vi "CRYUnflatten Display.vi"(11 "Flatten Display":string) -> (0 "Error?":bool=TRUE, 2 "DataView GUI Info":T1, 3 "Header info":T2={"Data type"="Data            ", "Version"=1, "Dimensions"=0})   [LabVIEW 2013]
uses:
  CRYWindow/DataView/VIEW/Control/Graph Main Info Cluster.ctl
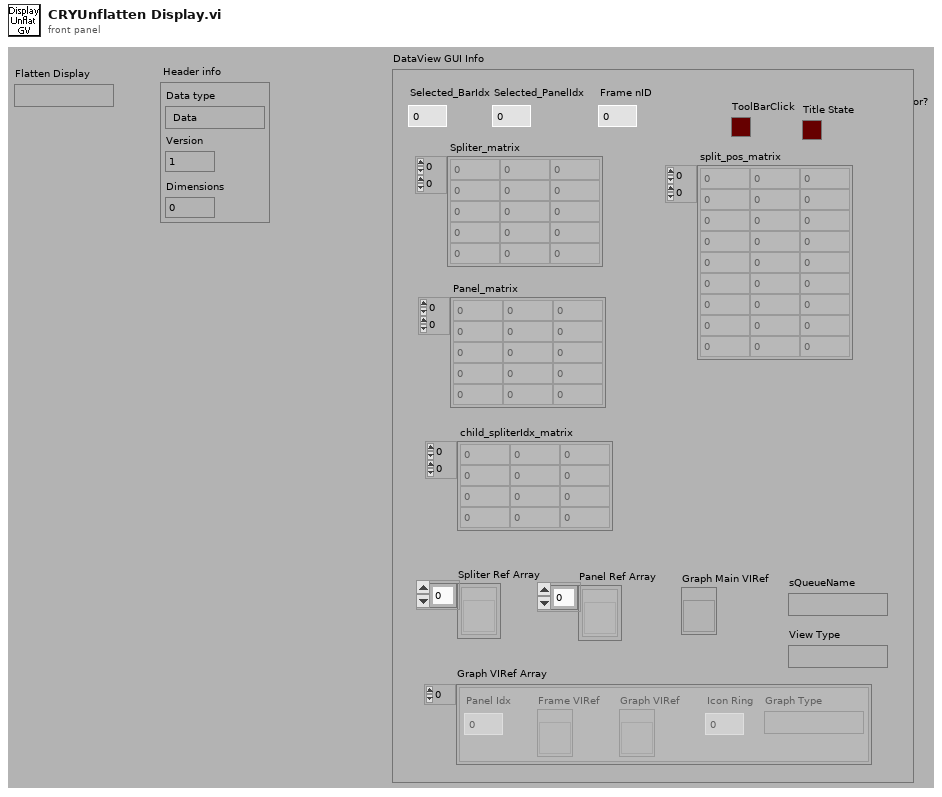
[diagram p1: front panel]
types:
  T1 = typedef "Graph Main Info Cluster.ctl" = cluster{"Selected_BarIdx":i32, "Selected_PanelIdx":i32, "Graph Main VIRef":refnum<vi>, "ToolBarClick":bool, "Spliter Ref Array":refnum<vi>[], "Panel Ref Array":refnum<vi>[], "Spliter_matrix":i32[][], "Panel_matrix":i32[][], "child_spliterIdx_matrix":i32[][], "split_pos_matrix":i32[][], "Title State":bool, "sQueueName":string, "Frame nID":i32, "Graph VIRef Array":cluster{"Graph VIRef":refnum<vi>, "Panel Idx":i32, "Frame VIRef":refnum<vi>, "Icon Ring":i32, "Graph Type":string}[], "View Type":string}
  T2 = cluster{"Data type":string, "Version":u16, "Dimensions":u8}
  T3 = cluster{"unsigned byte array[0]":u8, "unsigned byte array[1]":u8, "unsigned byte array[2]":u8}
  T4 = cluster{"substring":string, u16, "unsigned byte array[2]":u8}
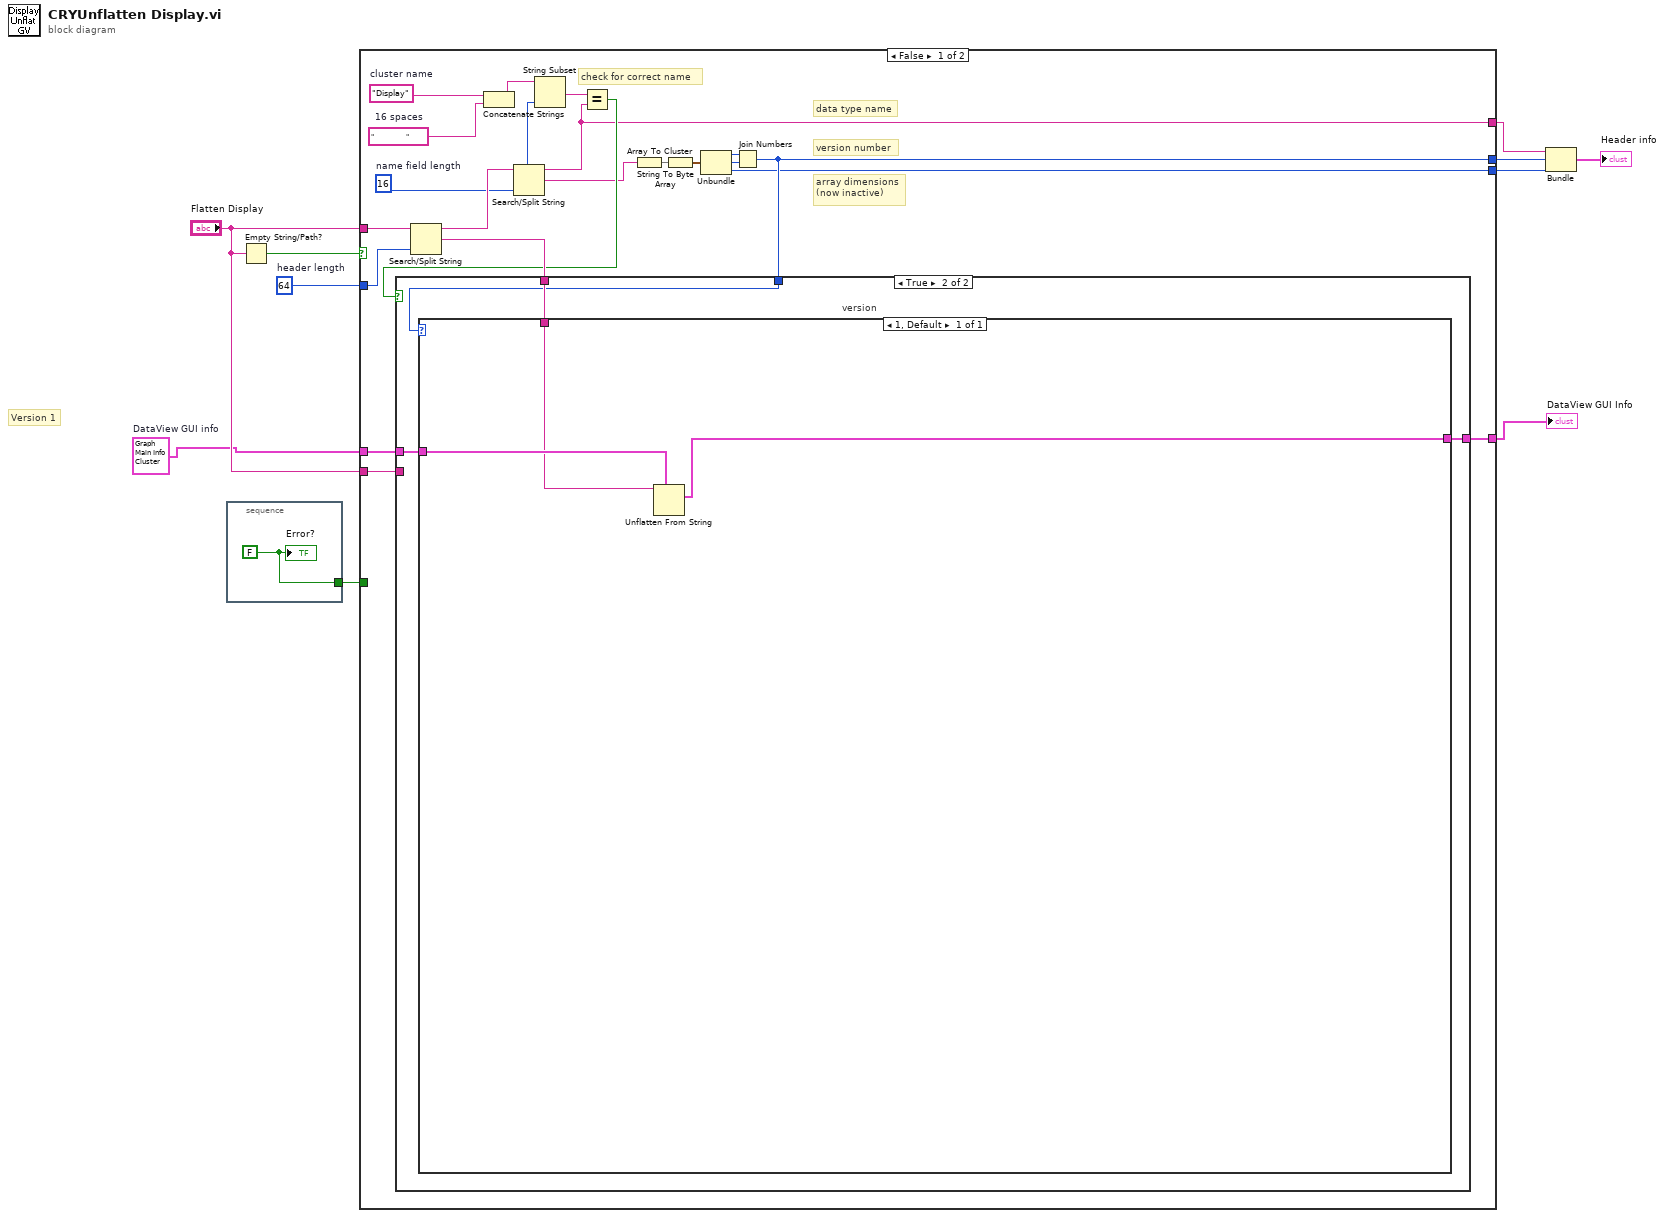
[diagram p0: block diagram]
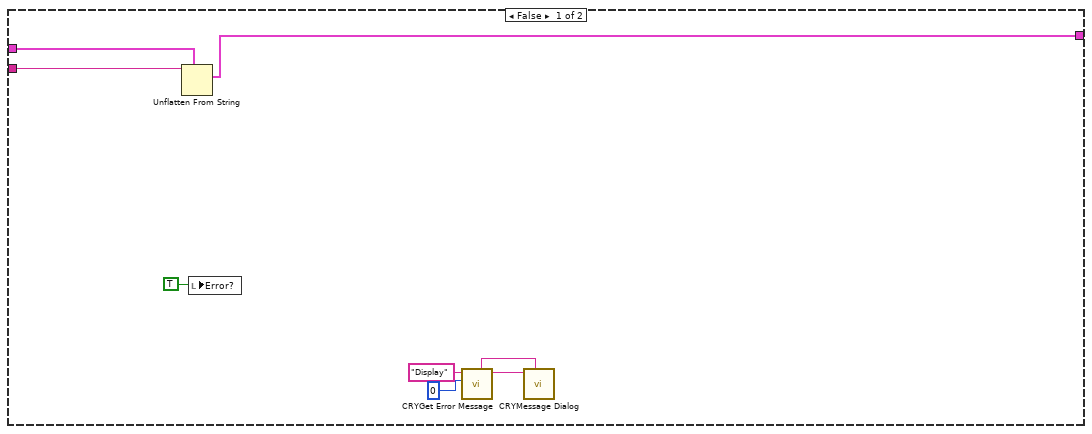
[diagram p2: hidden frame]
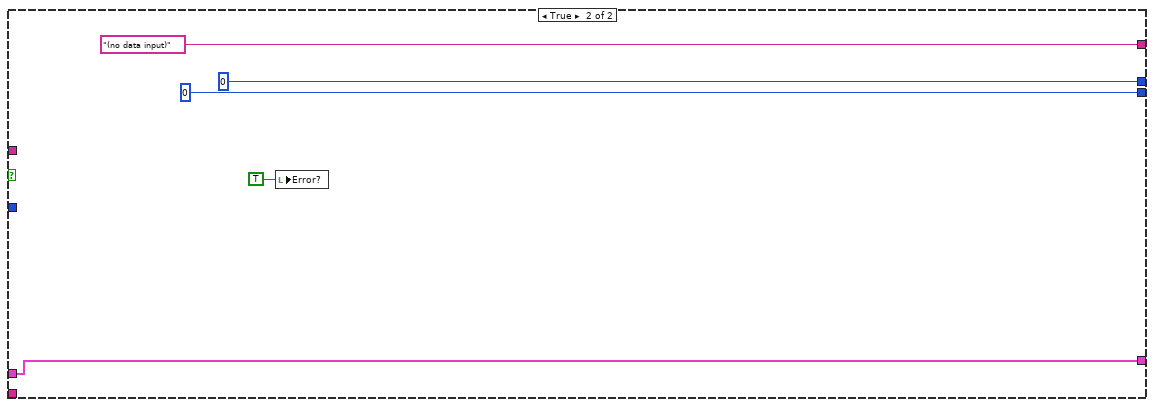
[diagram p3: hidden frame]
diagram:
  w2 = T1 {"Selected_BarIdx"=0, "Selected_PanelIdx"=0, "Graph Main VIRef"=refnum, "ToolBarClick"=FALSE, "Spliter Ref Array"=[], "Panel Ref Array"=[], "Spliter_matrix"=[], "Panel_matrix"=[], "child_spliterIdx_matrix"=[], "split_pos_matrix"=[], "Title State"=FALSE, "sQueueName"="", "Frame nID"=0, "Graph VIRef Array"=[], "View Type"=""}  # DataView GUI info
  w9 = 64  # header length
  # "Version 1"
  n1 = stacked-sequence {
    tunnel: [w11] -> w4
    frame #0 {
      w11 = FALSE
      "Error?" <- w11
    }
  }
  n2 = Empty String/Path?(string/path="Flatten Display") -> (empty?=w10:bool)
  n3 = case shown="False" w10 {
    tunnel: "Flatten Display" -> [w32 _]
    tunnel: w9 -> [w26 _]
    tunnel: [w23 u16 0] -> w7
    tunnel: [w15 u8 0] -> w8
    tunnel: [w16 "(no data input)" ("substring")] -> w6
    tunnel: w4 -> [_ _]
    tunnel: [w14 w48] -> w1
    tunnel: w2 -> [w13 w48]
    tunnel: "Flatten Display" -> [w12 _]
    frame False {
      w20 = "                "  # 16 spaces
      w21 = "Display"  # cluster name
      w18 = 16  # name field length
      # "check for correct name"
      # "array dimensions\n(now inactive)"
      # "version number"
      # "data type name"
      n4 = Search/Split String(string=w32, offset (0)=w26) -> (substring before match=w25:string, match + rest of string=w27:string)  [unwired: 2 out]
      n5 = Concatenate Strings(w21, w20) -> (w19:string)
      n6 = Search/Split String(string=w25, offset (0)=w18) -> (substring before match=w16:string, match + rest of string=w22:string)  [unwired: 2 out]
      n7 = String Subset(string=w19, length (rest)=w18) -> (substring=w17:string)  [unwired: 1 out]
      n8 = Equal?(x=w17, y=w16) -> (x = y?=w24:bool)
      n9 = String To Byte Array(string=w22) -> (unsigned byte array=w31:u8[])
      n10 = Array To Cluster(array=w31) -> (cluster=w30:T3)
      n11 = Unbundle(w30) -> ("unsigned byte array[0]"=w29:u8, "unsigned byte array[1]"=w28:u8, "unsigned byte array[2]"=w15:u8)
      n12 = Join Numbers(hi=w29, lo=w28) -> ((hi.lo)=w23:u16)
      n13 = case shown="True" w24 {
        tunnel: w27 -> [_ w44]
        tunnel: w23 -> [_ w43]
        tunnel: [w38 w41] -> w14
        tunnel: w13 -> [w39 w42]
        tunnel: w12 -> [w37 _]
        frame False {
          n14 = Unflatten From String(type=w39, binary string=w37) -> (value=w38:T1)  [unwired: 3 in, 2 out]
          n15 = local write "Error?"(TRUE) -> ()
          n16 = call "CRYGet Error Message.vi"("Error No"=0, "Kind"="Display") -> ("Message"=w34:string, "Window Title"=w33:string)  [unwired: 4 in, 4 out]
          n17 = call "CRYMessage Dialog.vi"("Window Title"=w33, "Message Content"=w34) -> ()  [unwired: 8 in, 2 out]
        }
        frame True {
          n18 = case "version" shown="1, Default" w43 {
            tunnel: w44 -> [w46]
            tunnel: w42 -> [w47]
            tunnel: [w45] -> w41
            frame 1, Default {
              n19 = Unflatten From String(type=w47, binary string=w46) -> (value=w45:T1)  [unwired: 3 in, 2 out]
            }
          }
        }
      }
    }
    frame True {
      n20 = local write "Error?"(TRUE ("Error?")) -> ()
    }
  }
  "DataView GUI Info" <- w1
  n21 = Bundle("substring"=w6, w7, "unsigned byte array[2]"=w8) -> (→"Header info":T4)  [unwired: 1 out]
